vi "Main.vi"() -> ()   [LabVIEW 2020]
doc: "This template is for the Queued Message Handler design pattern.\n\nThe Event Handling Loop generates messages based on user interface actions.\n\nThe Message Handling Loop processes messages generated by the Event Handling Loop, or by other messages. The messages are string values, so new messages can be added easily to the Message Cases case structure in the Message Handling Loop. Each message cluster can also provide an optional value for Message Data, which is a variant that can be converted to whatever message-specific data is required."
uses:
  controls/UI Data.ctl
  support/Message Queue/Message Cluster.ctl
  <vilib>/DAQmx/read.llb/DAQmx Read (Analog 1D DBL 1Chan NSamp).vi
  <extravilib>/ChannelInstances/Messenger-t'Message Queue.lvlib-Message Cluster.ctl'/Write With Abort.vi
  <extravilib>/ChannelInstances/Messenger-t'Message Queue.lvlib-Message Cluster.ctl'/Instantiate.vi
  <extravilib>/ChannelInstances/Messenger-t'Message Queue.lvlib-Message Cluster.ctl'/Endpoint.vi
  <extravilib>/ChannelInstances/Event Messenger-bool/Instantiate.vi
  <extravilib>/ChannelInstances/Event Messenger-bool/))Channel.vi
  <vilib>/DAQmx/create/channels.llb/DAQmx Create Channel (AI-Voltage-Basic).vi
  <vilib>/DAQmx/configure/timing.llb/DAQmx Timing (Sample Clock).vi
  <vilib>/DAQmx/miscellaneous.llb/DAQmx Fill In Error Info.vi
  <vilib>/Utility/error.llb/Error Cluster From Error Code.vi
  <vilib>/ErrorRing/Error Ring.xnode
  <extravilib>/ChannelInstances/Event Messenger-bool.lvlib
  support/Message Queue/Message Queue.lvlib
  <extravilib>/ChannelInstances/Messenger-t'Message Queue.lvlib-Message Cluster.ctl'.lvlib
  <resource>/objmgr/daqmx.rc
panel:
  out "Actual Sample Rate":dbl
  in  "Threshold":dbl=4.0
  in  "Analyze Signal":bool
  in  "Sample Rate":dbl=1000.0
  in  "Generate Signal":bool
  out "Threshold Exceeded?":bool
  out "RMS Result":dbl
  out "Current Consumer State":string
  out "Waveform Graph":dbl[](graph)
  in  "Exit":bool
  # "These controls have associated \"Value Changed\" events configured in the Event Structure on the diagram.\n\nReplace them (and reconfigure the Event Structure) with the controls you need for your application."
  # "This template is for the Queued Message Handler design pattern.\n\nSee the block diagram for more information on how to use this template."
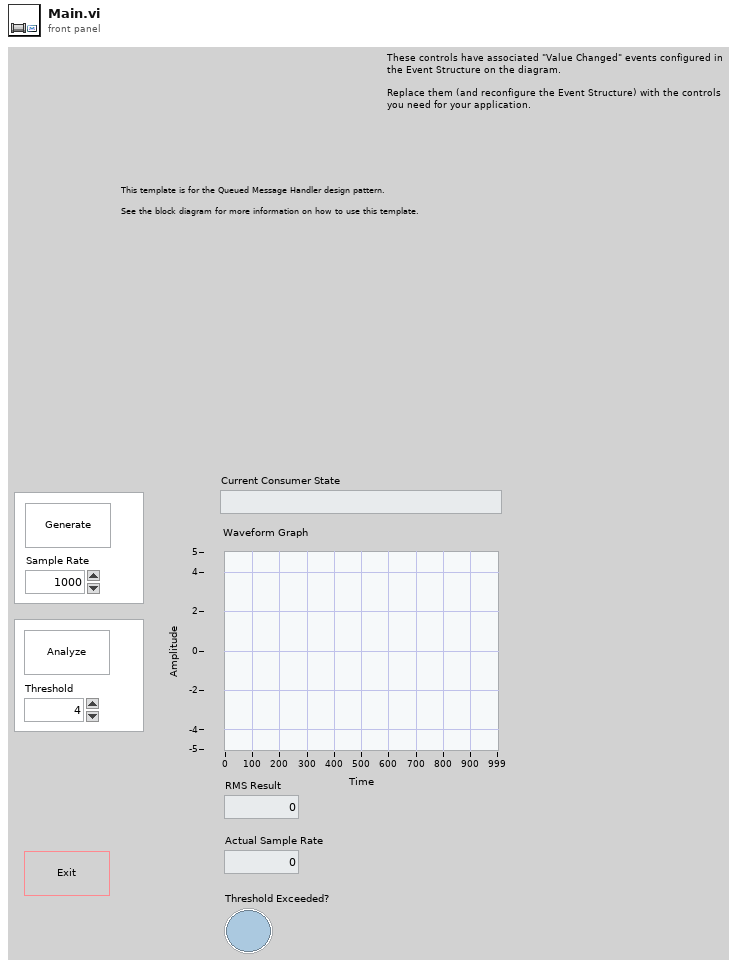
[diagram p1: front panel]
types:
  T1 = typedef "Message Queue.lvlib/Message Cluster.ctl" = cluster{"Message":string, "Message Data":variant}
  T2 = typedef "UI Data.ctl" = cluster{"Message":string, "Message Data":u32}
  T3 = typedef "Messenger-t'Message Queue.lvlib-Message Cluster.ctl'.lvlib/))Channel.ctl" = refnum<queue>
  T4 = typedef "Event Messenger-bool.lvlib/))Channel.ctl" = refnum<queue>
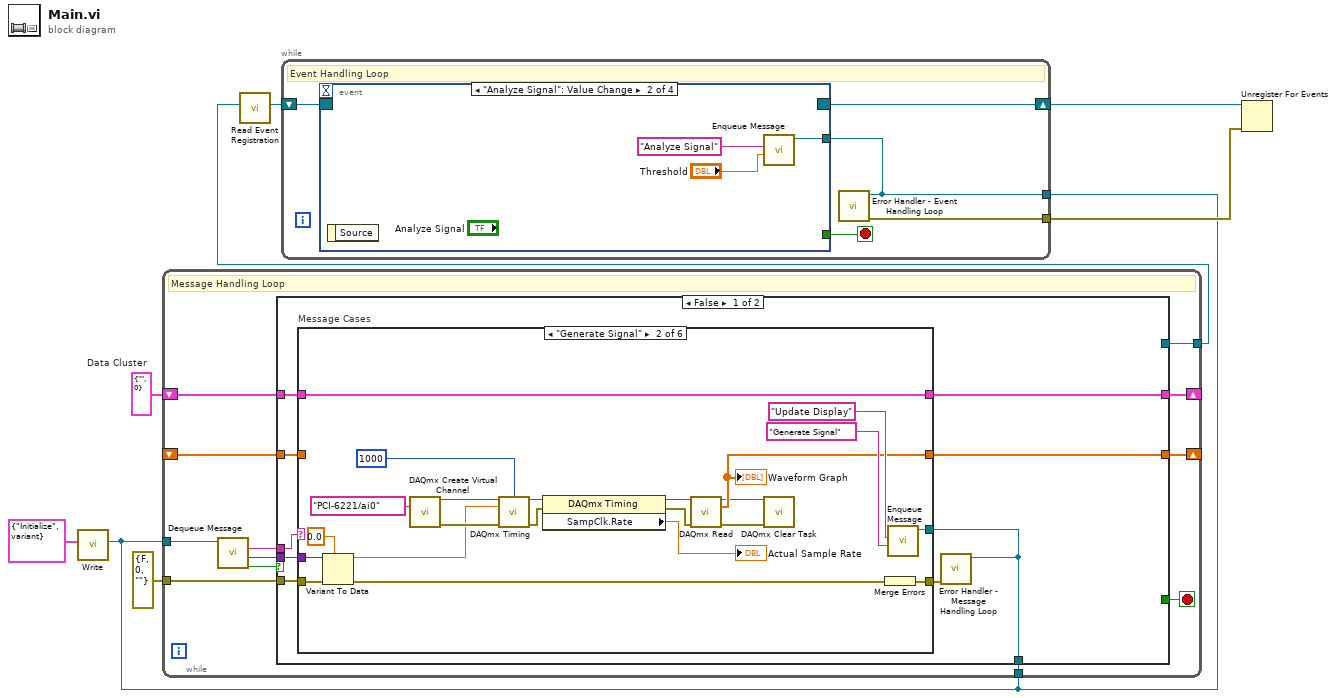
[diagram p0: block diagram]
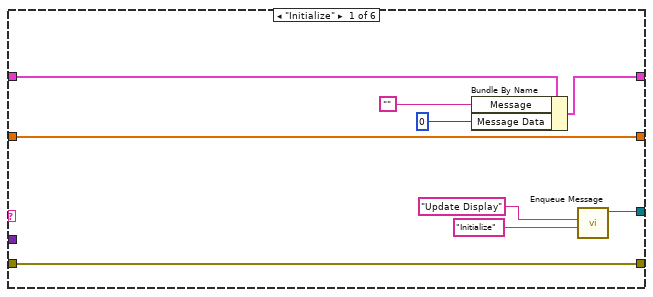
[diagram p2: hidden frame]
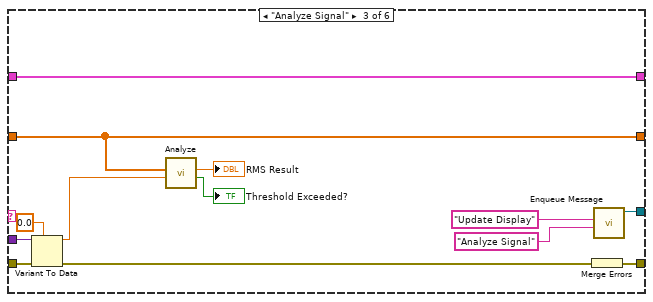
[diagram p3: hidden frame]
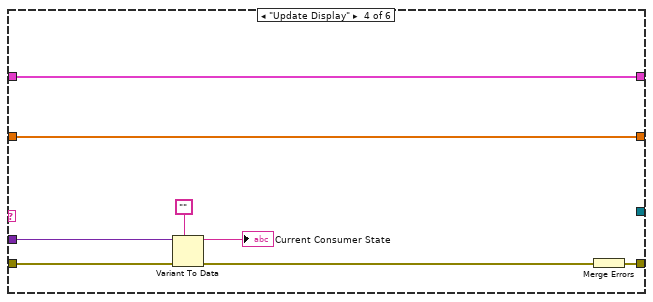
[diagram p4: hidden frame]
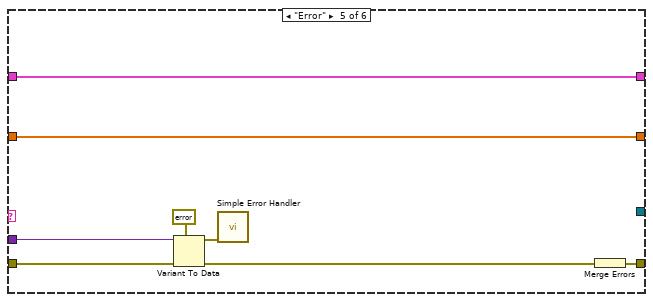
[diagram p5: hidden frame]
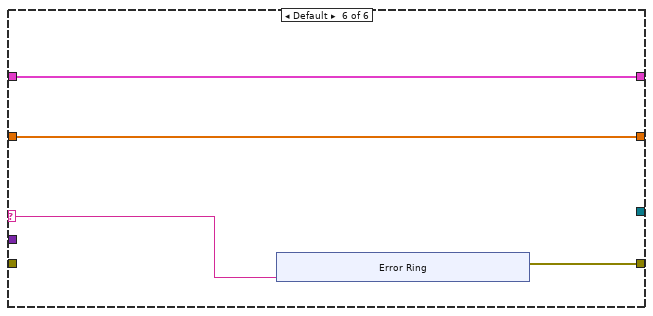
[diagram p6: hidden frame]
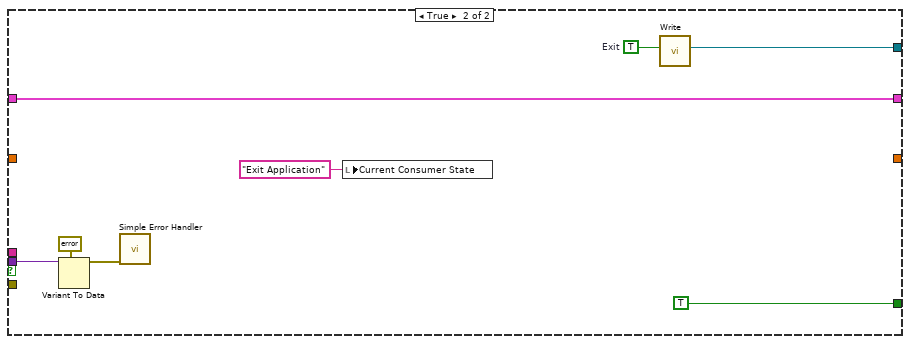
[diagram p7: hidden frame]
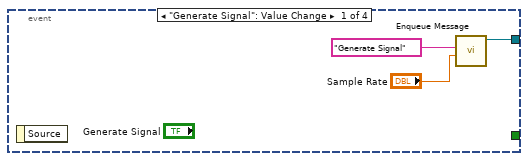
[diagram p8: hidden frame]
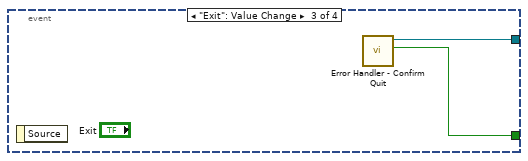
[diagram p9: hidden frame]
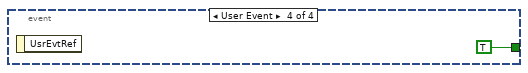
[diagram p10: hidden frame]
diagram:
  w7 = T2 {"Message"="", "Message Data"=0}  # Data Cluster
  n1 = call <extravilib>:"Write.vi"("element"=T1 {"Message"="Initialize", "Message Data"=variant}) -> ("channel"=w2:T3)  [unwired: 8 in, 2 out]
  n2 = while {
    shift-right: [w19] -> _
    shift-left: w7 -> [w20]
    tunnel: [w17] -> w5
    tunnel: w2 -> [w14]
    tunnel: errorcluster {"status"=FALSE, "code"=0, "source"=""} ("error IO") -> [w16]
    tunnel: w2 -> [w15]
    shift-right: [w10] -> _
    shift-left: _ -> [w9]
    stop <- w18 stop-if-true
    # "Message Handling Loop"
    n3 = call "Dequeue Message.vi"("channel"=w14) -> ("channel aborted"=w11:bool, "message data"=w12:variant, "message"=w13:string)  [unwired: 8 in]
    n4 = case shown="False" w11 {
      tunnel: w20 -> [w29 w107]
      tunnel: [w28 w107] -> w19
      tunnel: [_ TRUE] -> w18
      tunnel: [_ w102] -> w17
      tunnel: w13 -> [w26 _]
      tunnel: w12 -> [w25 w104]
      tunnel: w16 -> [w24 _]
      tunnel: [w23 _] -> w15
      tunnel: [w22 _] -> w10
      tunnel: w9 -> [w21 _]
      frame False {
        n5 = case "Message Cases" shown="\"Generate Signal\"" w26 {
          selector: w26 -> [_ _ _ _ _ w91]
          tunnel: w24 -> [w36 w46 w65 w79 w89 _]
          tunnel: [w36 w59 w72 w80 w83 w92] -> w27
          tunnel: w29 -> [w38 w60 w73 w81 w88 w93]
          tunnel: [w37 w60 w73 w81 w88 w93] -> w28
          tunnel: w25 -> [_ w48 w64 w78 w87 _]
          tunnel: [w33 w58 w71 _ _ _] -> w23
          tunnel: [w30 w55 w67 w75 w82 w90] -> w22
          tunnel: w21 -> [w30 _ w67 w75 w82 w90]
          frame "Initialize" {
            # "Initialize - All initialization work should take place in this message, since other loops can potentially enqueue messages that execute immediately after this one."
            n6 = Bundle By Name(cluster=w38, "Message"="", "Message Data"=u32 0 ("Numeric <Replace Me>")) -> (w37:T2)
            n7 = call "Enqueue Message.vi"("data (empty)"="Initialize" ("Initial Message"), "message"="Update Display" ("Message")) -> ("channel"=w33:T3)  [unwired: 9 in]
          }
          frame "Generate Signal" {
            # "Something - Replace this message with functionality for your own application."
            n8 = Variant To Data(error in=w46, type=0.0, Variant=w48) -> (data=w44:dbl, error out=w45:errorcluster)
            n9 = call-poly <vilib>:"DAQmx Create Virtual Channel.vi"("physical channels"=tag "PCI-6221/ai0") -> ("task out"=w54:refnum<k21>, "error out"=w53:errorcluster)  [unwired: 13 in]
            n10 = call-poly <vilib>:"DAQmx Timing.vi"("task/channels in"=w54, "samples per channel"=1000, "rate"=w44, "error in"=w53) -> ("task out"=w43:refnum<k21>, "error out"=w42:errorcluster)  [unwired: 10 in]
            n11 = property class="DAQmx Timing"(reference=w43, error in=w42) -> (reference out=w41:refnum<k21>, error out=w40:errorcluster, "SampClk.Rate"=→"Actual Sample Rate":dbl)
            n12 = call-poly <vilib>:"DAQmx Read.vi"("task/channels in"=w41, "error in"=w40) -> ("task out"=w52:refnum<k21>, "data"=w55:dbl[], "error out"=w51:errorcluster)  [unwired: 11 in]
            "Waveform Graph" <- w55
            n13 = call <vilib>:"DAQmx Clear Task.vi"("task in"=w52, "error in"=w51) -> ()  [unwired: 13 in, 1 out]
            n14 = Merge Errors(w45) -> (w59:errorcluster)
            n15 = call "Enqueue Message.vi"("data (empty)"="Generate Signal" ("\"Do Something\" button pressed"), "message"="Update Display" ("Message")) -> ("channel"=w58:T3)  [unwired: 9 in]
          }
          frame "Analyze Signal" {
            # "Something Else - Replace this message with functionality for your own application."
            n16 = Variant To Data(error in=w65, type=0.0, Variant=w64) -> (data=w62:dbl, error out=w63:errorcluster)
            n17 = call "Analyze.vi"("Threshold (rms)"=w62, "Data (1D DBL)"=w67) -> ("Threshold Exceeded?"=→"Threshold Exceeded?":bool, "RMS Result"=→"RMS Result":dbl)  [unwired: 8 in]
            n18 = Merge Errors(w63) -> (w72:errorcluster)
            n19 = call "Enqueue Message.vi"("data (empty)"="Analyze Signal" ("\"Do Something Else\" button pressed"), "message"="Update Display" ("Message")) -> ("channel"=w71:T3)  [unwired: 9 in]
          }
          frame "Update Display" {
            # "Update Display - Convert the message data to a string to display in the Data Display indicator."
            n20 = Variant To Data(error in=w79, type="", Variant=w78) -> (data=→"Current Consumer State":string, error out=w76:errorcluster)
            n21 = Merge Errors(w76) -> (w80:errorcluster)
          }
          frame "Error" {
            # "Error - Display an error dialog. This message is sent by the \"Error Handler\" VIs at the end of other loops in this application."
            n22 = Variant To Data(error in=w89, type=errorcluster {"status"=FALSE, "code"=0, "source"=""} ("error constant"), Variant=w87) -> (data=w85:errorcluster, error out=w84:errorcluster)
            n23 = call <vilib>:"Simple Error Handler.vi"("error in (no error)"=w85) -> ()  [unwired: 4 in, 5 out]
            n24 = Merge Errors(w84) -> (w83:errorcluster)
          }
          frame Default {
            # "'Default' case only runs if there is a message that isn't defined in any of the other cases.  Output a programming error."
            n25 = xnode "Error Ring"("parameter 0"=w91) -> ("error out"=w92:errorcluster)
          }
        }
        n26 = call "Error Handler - Message Handling Loop.vi"("channel"=w23, "error in (no error)"=w27) -> ()  [unwired: 9 in, 1 out]
      }
      frame True {
        w103 = TRUE  # Exit
        n27 = Variant To Data(type=errorcluster {"status"=FALSE, "code"=0, "source"=""} ("error constant"), Variant=w104) -> (data=w105:errorcluster)  [unwired: 1 in, 1 out]
        n28 = call <vilib>:"Simple Error Handler.vi"("error in (no error)"=w105) -> ()  [unwired: 4 in, 5 out]
        n29 = local write "Current Consumer State"("Exit Application" ("Exit Application")) -> ()
        n30 = call <extravilib>:"Write.vi"("element"=w103) -> ("channel"=w102:T4)  [unwired: 9 in, 1 out]
      }
    }
  }
  n31 = call <extravilib>:"Read Event Registration.vi"("channel"=w5) -> ("event registration refnum"=w4:refnum<event-registration>)  [unwired: 10 in]
  n32 = while {
    shift-right: [w112] -> w8
    shift-left: w4 -> [w113]
    tunnel: [w110] -> w6
    tunnel: w2 -> [w109]
    stop <- w111 stop-if-true
    # "Event Handling Loop"
    n33 = event shown="[1] \"Analyze Signal\": Value Change" {
      selector: w113 -> [_ _ _ _]
      dyn-events: [_ _ _ _] -> w112
      timeout: _ -> [_ _ _ _]
      tunnel: [_ _ w120 TRUE ("Discard?")] -> w111
      tunnel: [w116 w119 w121 _] -> w109
      event "Generate Signal": Value Change {
        n34 = event-data() -> ()  [unwired: 1 in, 1 out]
        n35 = call "Enqueue Message.vi"("data (empty)"="Sample Rate", "message"="Generate Signal" ("Message")) -> ("channel"=w116:T3)  [unwired: 9 in]
      }
      event "Analyze Signal": Value Change {
        n36 = event-data() -> ()  [unwired: 1 in, 1 out]
        n37 = call "Enqueue Message.vi"("data (empty)"="Threshold", "message"="Analyze Signal" ("Message")) -> ("channel"=w119:T3)  [unwired: 9 in]
      }
      event "Exit": Value Change {
        n38 = event-data() -> ()  [unwired: 1 in, 1 out]
        n39 = call "Error Handler - Confirm Quit.vi"() -> ("exit confirmed"=w120:bool, "channel"=w121:T3)  [unwired: 10 in]
      }
      event User Event {
        n40 = event-data() -> ()  [unwired: 1 in, 1 out]
      }
    }
    n41 = call "Error Handler - Event Handling Loop.vi"("channel"=w109) -> ("dup error in"=w110:errorcluster)  [unwired: 10 in]
  }
  n42 = Unregister For Events(event registration refnum=w8, error in=w6) -> ()  [unwired: 1 out]
